vi "CANOpen Add TPDO.vi"(8 "error in (no error)":errorcluster, 11 "Node Ptr":u64 format="%.0x") -> (0 "error out":errorcluster)   [LabVIEW 2013, in "CANOpen Addon Custom Device.lvlib"]
uses:
  CANOpen Addon Custom Device.lvlib
  SubVIs/CANOpen_PDO Type.ctl
panel:
  in  "Tag":string
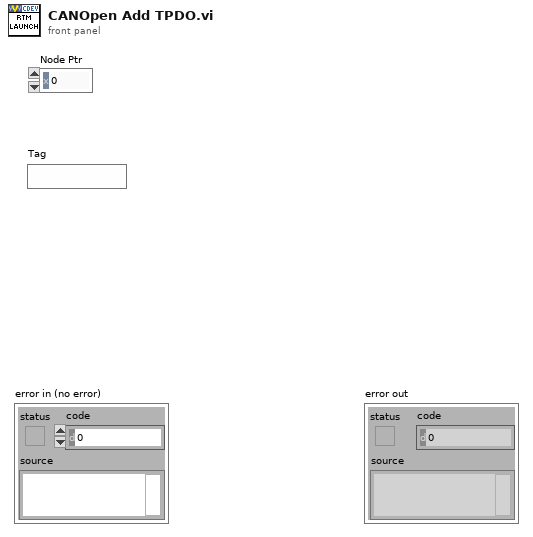
[diagram p1: front panel]
types:
  T1 = typedef "CANOpen_PDO Type.ctl" = enum16{"RPDO", "TPDO"}
  T2 = typedef "CANOpen Addon Custom Device.lvlib/CANOpen_PDO Settings.ctl" = cluster{"Parameters":T3[], "PDO Channel":u8, "Start Index":u32, "Length":u32}
  T3 = typedef "CANOpen Addon Custom Device.lvlib/CANOpen_PDO Parameter Settings.ctl" = cluster{"Parameter Name":string, "Scale Factor":dbl, "Scale Offset":dbl, "Byte Offset":u8, "Bit Offset":u8, "Data Type":T4, "Byte Order":T5}
  T4 = typedef "CANOpen Addon Custom Device.lvlib/CANOpen_PDO Data Type.ctl" = enum16{"U8", "U16", "U32", "I8", "I16", "I32", "Single", "Double", "Boolean"}
  T5 = typedef "CANOpen Addon Custom Device.lvlib/CANopen Byte Order.ctl" = enum16{"big-endian network order", "little-endian"}
  T6 = typedef "Custom Device API.lvlib/Custom Device Item Ref.ctl" = u64
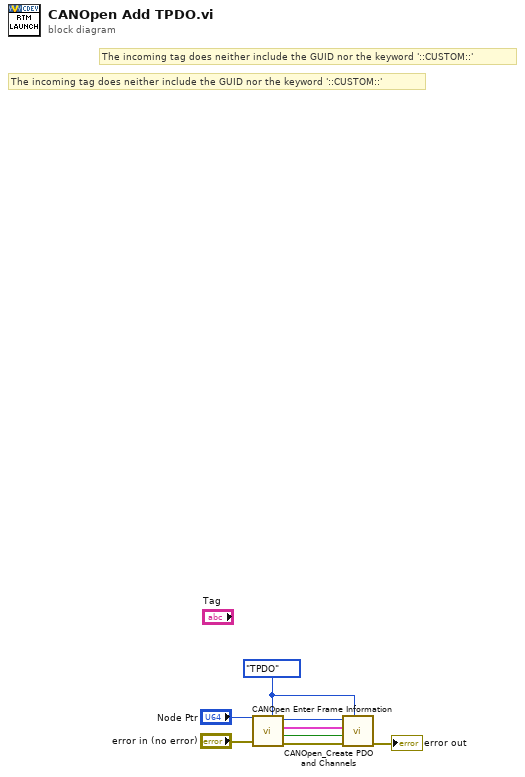
[diagram p0: block diagram]
diagram:
  w1 = CANOpen_PDO_Type."TPDO" ("Type")
  # "The incoming tag does neither include the GUID nor the keyword '::CUSTOM::'"
  # "The incoming tag does neither include the GUID nor the keyword '::CUSTOM::'"
  n1 = call "CANOpen Enter Frame Information.vi"("Type"=w1, "error in (no error)"="error in (no error)", "Node Ptr"="Node Ptr") -> ("error out"=w7:errorcluster, "Cancelled?"=w2:bool, "PDO Settings"=w3:T2, "Item Ref out"=w8:T6)  [unwired: 5 in]
  n2 = call "CANOpen_Create PDO and Channels.vi"("Type"=w1, "error in (no error)"=w7, "Cancelled?"=w2, "PDO Settings"=w3, "Item Ref out"=w8) -> ("error out"=→"error out":errorcluster)  [unwired: 5 in, 1 out]
